vi "Generate Event to View.vi"(8 "error in":errorcluster, 9 "Event":refnum<class "Event.lvclass">, 10 "View Name":string, 11 "Controller In":refnum<class "Controller.lvclass">) -> (0 "error out":errorcluster, 3 "Controller Out":refnum<class "Controller.lvclass">)   [LabVIEW 2023, in "MVC Actors.lvlib" / "Controller.lvclass"]
doc: "Generates the event <b>Event</b> to the View Actor with name <b>View Name</b>. This is typically used in the overridden method \"Finalize View Init.vi\" to init a specific View Actor upon its launch."
uses:
  Controller.lvclass
  Event/Event.lvclass
  Controller.lvclass/Controller.ctl
  Event Handler Details.ctl
  Event Handlers/Abstract Event Message for View/Abstract Event Message for View.lvclass
  C:/Program Files/National Instruments/LabVIEW 2023/vi.lib/ActorFramework/Message/Message.lvclass
  Event Handlers/Abstract Event Message for View/Abstract Event Message for View.lvclass/Abstract Event Message for View.ctl
  <vilib>/ActorFramework/Message Enqueuer/Message Enqueuer.lvclass/Message Enqueuer.ctl
  Event Handlers/Abstract Event Message for View/Send Abstract Event Message for View.vi
  <vilib>/Utility/error.llb/Clear Errors.vi
  <vilib>/ActorFramework/Message Enqueuer/Enqueue.vi
  <vilib>/Utility/LVClass/Get LV Class Name.vi
  <resource>/AFDebug/Generate Trace for Message.vi
  <vilib>/ActorFramework/Message Priority Queue/Priority Enqueue.vi
  <vilib>/ActorFramework/Message Enqueuer/Message Enqueuer.lvclass
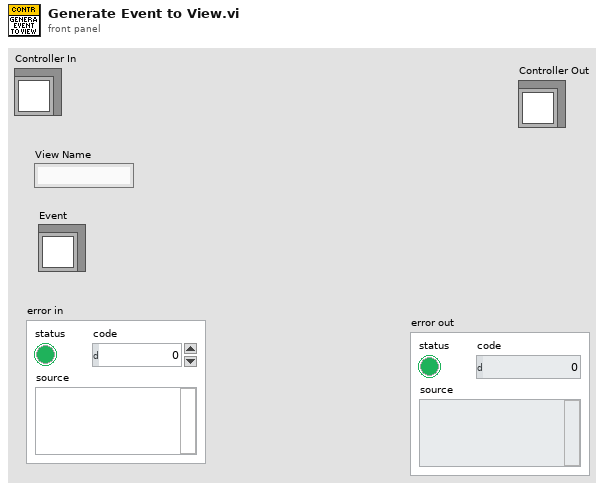
[diagram p1: front panel]
types:
  T1 = typedef "MVC Actors.lvlib/Controller.lvclass/View Details.ctl" = cluster{"Exclude From Broadcast":bool, "Receive Only":bool, "Paused":bool, "View Enqueuer":refnum<class "Message Enqueuer.lvclass">}
  T2 = typedef "MVC Actors.lvlib/Controller.lvclass/Event Handler Details.ctl" = cluster{"Exclude From Broadcast":bool, "Paused":bool, "View Event Fire Handler":refnum<class "Abstract Event Message for View.lvclass">}
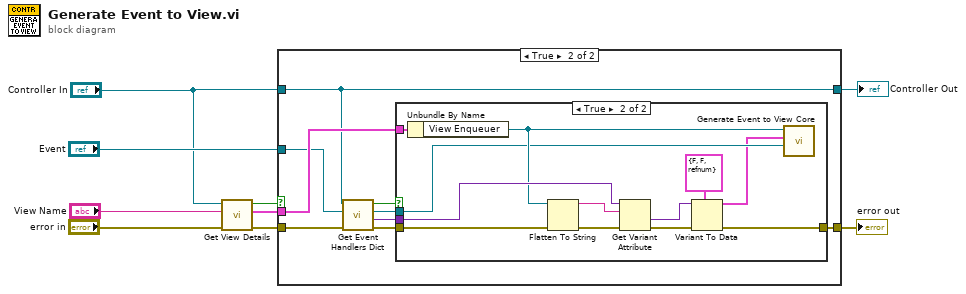
[diagram p0: block diagram]
diagram:
  n1 = call "Get View Details.vi"("error in (no error)"="error in", "View Name"="View Name", "Controller Actor in"="Controller In") -> ("error out"=w5:errorcluster, "View Details"=w7:T1, "View Found"=w2:bool)  [unwired: 6 in]
  n2 = case shown="True" w2 {
    tunnel: w7 -> [_ w20]
    tunnel: "Event" -> [_ w18]
    tunnel: w5 -> [w10 w16]
    tunnel: [w10 w14] -> w4
    tunnel: "Controller In" -> [w11 w13]
    tunnel: [w11 w13] -> w1
    frame False {
    }
    frame True {
      n3 = call "Get Event Handlers Dict.vi"("error in (no error)"=w16, "Event In"=w18, "Controller Actor in"=w13) -> ("error out"=w15:errorcluster, "Event Handlers Dict"=w19:variant, "Event out"=w17:refnum<class "Event.lvclass">, "Event Found"=w12:bool)  [unwired: 4 in, 1 out]
      n4 = case shown="True" w12 {
        tunnel: w20 -> [_ w33]
        tunnel: w19 -> [_ w32]
        tunnel: w17 -> [_ w27]
        tunnel: w15 -> [w21 w24]
        tunnel: [w21 w22] -> w14
        frame False {
        }
        frame True {
          n5 = Unbundle By Name(w33) -> ("View Enqueuer"=w31:refnum<class "Message Enqueuer.lvclass">)
          n6 = Flatten To String(anything=w31, error in (no error)=w24) -> (data string=w30:string, error out=w25:errorcluster)  [unwired: 2 in, 1 out]
          n7 = Get Variant Attribute(Variant=w32, name=w30, error in=w25) -> (value=w28:variant, error out=w23:errorcluster)  [unwired: 1 in, 2 out]
          n8 = Variant To Data(error in=w23, type=T2 {"Exclude From Broadcast"=FALSE, "Paused"=FALSE, "View Event Fire Handler"=refnum} ("Message Type"), Variant=w28) -> (data=w26:T2, error out=w22:errorcluster)
          n9 = call "Generate Event to View Core.vi"("Event in"=w27, "Event Handler Details"=w26, "Message Enqueuer in"=w31) -> ()  [unwired: 9 in]
        }
      }
    }
  }
  "error out" <- w4
  "Controller Out" <- w1
